vi "GEA2 Script_Verify GEA2 Responses.vi"(0 "Actual Response":T1 {"CRC" format="%04x"; "Length" format="%02x"; "Command" format="%02x"; "Destination" format="%02x"; "Source" format="%02x"}, 7 "Expected Response":string, 11 "Error In":errorcluster) -> (4 "Pass/Fail?":bool, 6 "Report Text":string, 15 "Error Out":errorcluster)   [LabVIEW 2023]
doc: "This parses all GEA2 responses and verifies them the expected messages. This VI always verifies that the total # of messages received matches the expected number."
uses:
  LabVIEW GEA2 Toolkit/GEA3/type defs/Data Out.ctl
  LabVIEW GEA2 Toolkit/GEA3/library/GEA2_Toolkit.lvlib
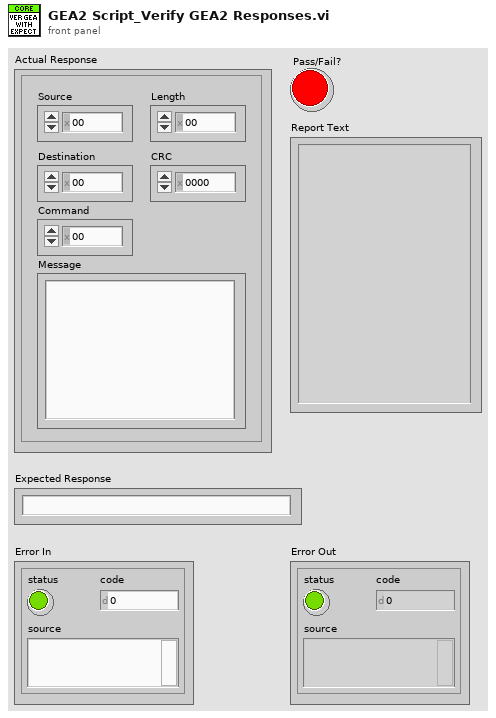
[diagram p1: front panel]
types:
  T1 = typedef "GEA2_Toolkit.lvlib/Data Out.ctl" = cluster{"Source":u8, "Destination":u8, "Command":u8, "Length":u8, "CRC":u16, "Message":string}
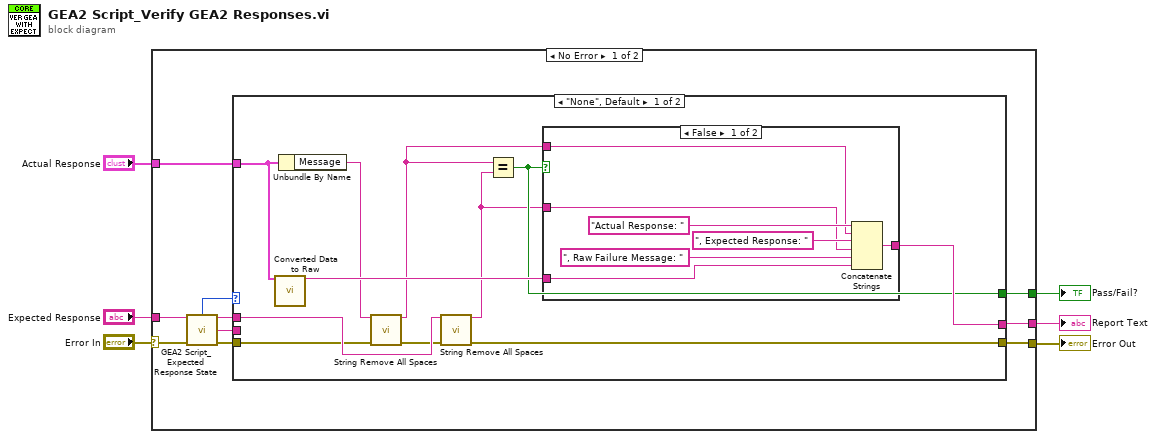
[diagram p0: block diagram]
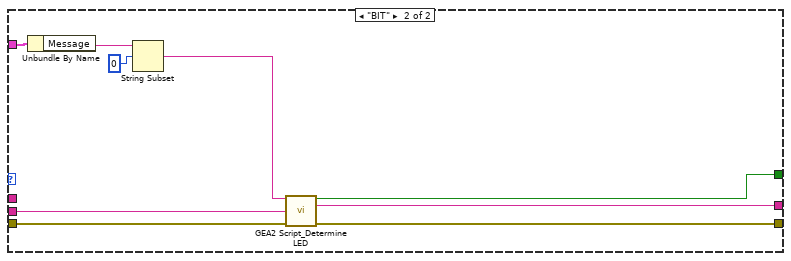
[diagram p3: hidden frame]
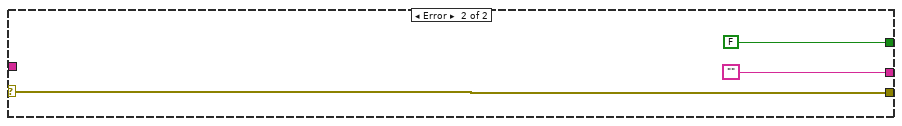
[diagram p4: hidden frame]
diagram:
  n1 = case shown="No Error" "Error In" {
    selector: "Error In" -> [w16 w44]
    tunnel: "Expected Response" -> [w7 _]
    tunnel: [w10 ""] -> w6
    tunnel: [w9 FALSE] -> w5
    tunnel: [w15 w44] -> w3
    tunnel: "Actual Response" -> [w8 _]
    frame No Error {
      n2 = call "GEA2 Script_Expected Response State.vi"("Expected Response In"=w7, "Error In"=w16) -> ("Response State"=w14:enum16{"None", "BIT"}, "Expected Response Out"=w12:string, "Match Substring"=w11:string, "Error Out"=w13:errorcluster)  [unwired: 10 in]
      n3 = case shown="\"None\", Default" w14 {
        tunnel: w8 -> [w27 w43]
        tunnel: [w25 w35] -> w10
        tunnel: [w24 w36] -> w9
        tunnel: w13 -> [w17 w40]
        tunnel: [w20 w38] -> w15
        tunnel: w12 -> [w21 _]
        tunnel: w11 -> [_ w39]
        frame "None", Default {
          n4 = call "Converted Data to Raw.vi"("Data In"=w27) -> ("Raw Data Out"=w26:string)  [unwired: 13 in, 1 out]
          n5 = Unbundle By Name(w27) -> ("Message"=w23:string)
          n6 = call "String Remove All Spaces.vi"("Input String"=w23, "error in (no error)"=w17) -> ("Spaces Removed"=w22:string, "error out"=w18:errorcluster)  [unwired: 12 in]
          n7 = call "String Remove All Spaces.vi"("Input String"=w21, "error in (no error)"=w18) -> ("Spaces Removed"=w19:string, "error out"=w20:errorcluster)  [unwired: 12 in]
          n8 = Equal?(x=w22, y=w19) -> (x = y?=w24:bool)
          n9 = case shown="False" w24 {
            tunnel: w19 -> [w30 _]
            tunnel: w22 -> [w31 _]
            tunnel: w26 -> [w29 _]
            tunnel: [w28 _] -> w25
            frame False {
              n10 = Concatenate Strings("Actual Response: " ("string"), w31, ", Expected Response: " ("string"), w30, ", Raw Failure Message: " ("string"), w29) -> (w28:string)
            }
            frame True {
            }
          }
        }
        frame "BIT" {
          n11 = Unbundle By Name(w43) -> ("Message"=w37:string)
          n12 = String Subset(string=w37, offset (0)=0) -> (substring=w41:string)  [unwired: 1 in]
          n13 = call "GEA2 Script_Determine LED.vi"("LED Data In"=w41, "Match Substring In"=w39, "Error In"=w40) -> ("Pass/Fail?"=w36:bool, "Report Text"=w35:string, "Error Out"=w38:errorcluster)  [unwired: 10 in]
        }
      }
    }
    frame Error {
    }
  }
  "Report Text" <- w6
  "Pass/Fail?" <- w5
  "Error Out" <- w3
